vi "Get Behavior Flags.vi"(8 "error in (no error)":errorcluster, 11 "Attribute in":refnum<class "Attribute.lvclass">) -> (0 "error out":errorcluster, 2 "Behavior":T1={"Children"=enum."One", "Editable"=TRUE, "XML uses />"=FALSE}, 3 "Attribute out":refnum<class "Attribute.lvclass">)   [LabVIEW 2026, in "VILab.lvlib" / "Attribute.lvclass"]
uses:
  Attribute.lvclass
  Data Item/Behavior Flags.ctl
  Data Item/Child Support.ctl
  Data Item/Data Item.lvclass
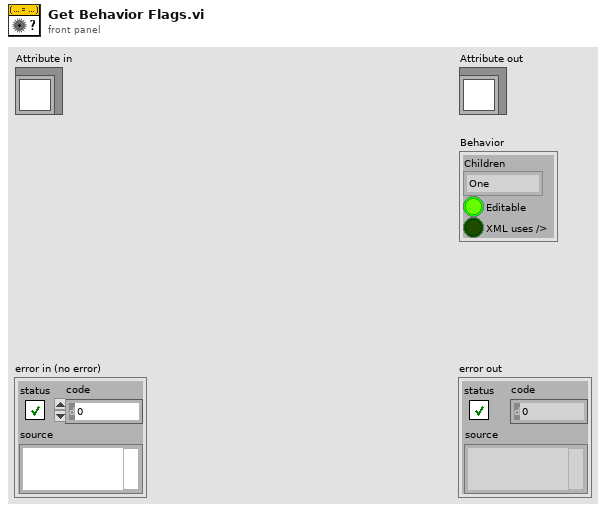
[diagram p1: front panel]
types:
  T1 = typedef "VILab.lvlib/Data Item.lvclass/Behavior Flags.ctl" = cluster{"Children":T2, "Editable":bool, "XML uses />":bool}
  T2 = typedef "VILab.lvlib/Data Item.lvclass/Child Support.ctl" = enum16{"None", "One", "At most one", "Multiple"}
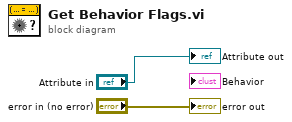
[diagram p0: block diagram]
diagram:
  "error out" <- "error in (no error)"
  "Attribute out" <- "Attribute in"
